vi "0814 labviewToEsp32.vi"(0 "power step  4":string, 1 "power step  3":string, 2 "power step  2":string, 3 "power step  1":string, 5 "power step  5":string, 6 "direction":string, 8 "scanspeed (um/s)":string, 9 "count":string, 10 "um":string, 11 "Ring":u16(ring) items=["Move X"=1, "Move Y"=2, "Single shot"=3, "single shot *15"=4, "energy adjustment"=5, "knife edge method"=6, "Auto mode"=7, "multiple shot"=8, "power change"=9, "shutter+move"=10, "stop"=0]) -> (4 "output":string)   [LabVIEW 2018]
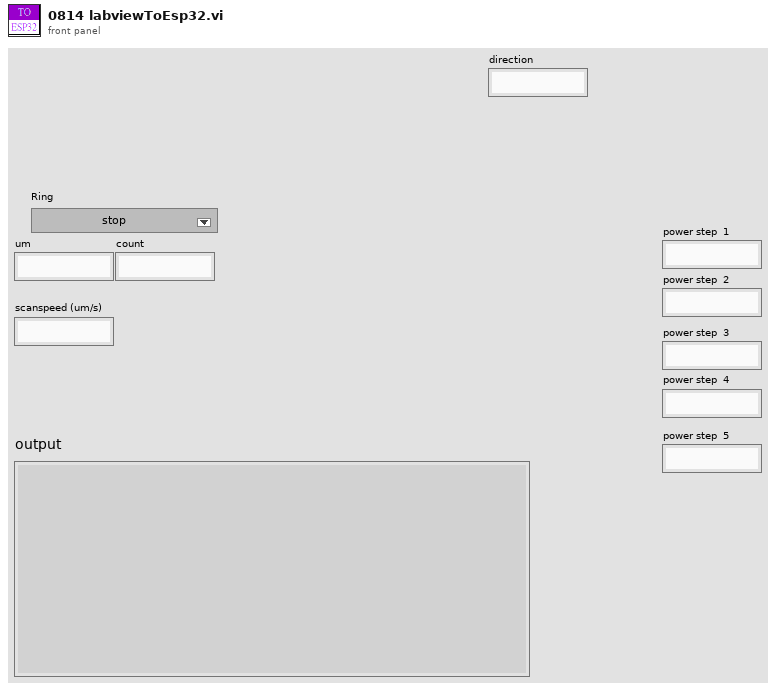
[diagram p1: front panel]
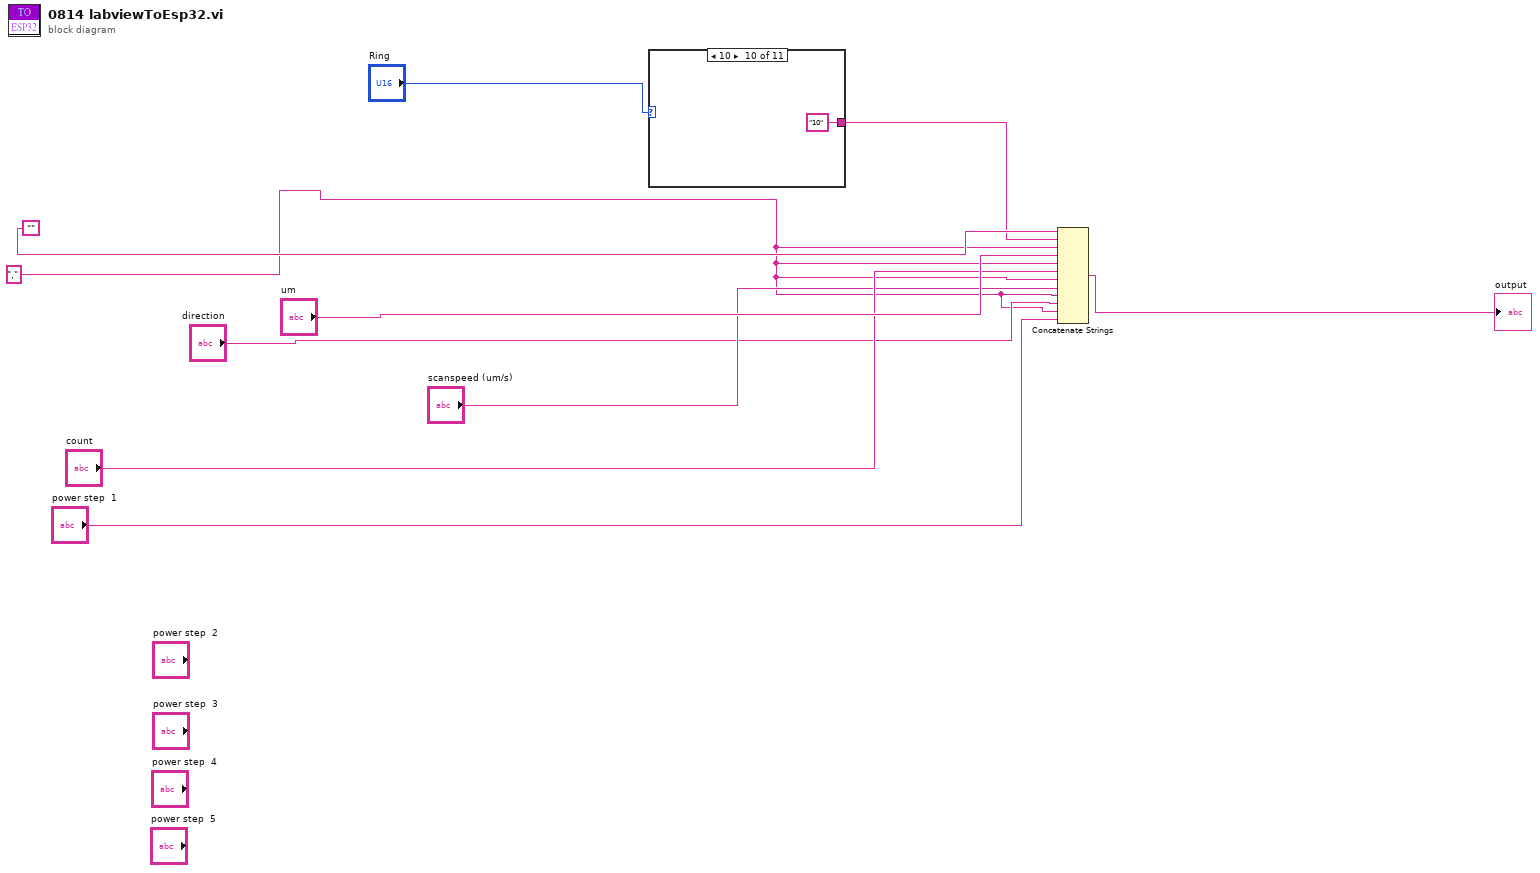
[diagram p0: block diagram]
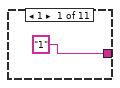
[diagram p2: hidden frame]
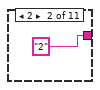
[diagram p3: hidden frame]
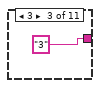
[diagram p4: hidden frame]
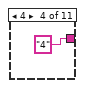
[diagram p5: hidden frame]
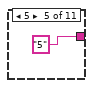
[diagram p6: hidden frame]
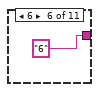
[diagram p7: hidden frame]
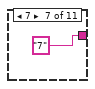
[diagram p8: hidden frame]
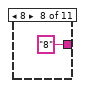
[diagram p9: hidden frame]
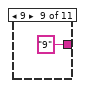
[diagram p10: hidden frame]
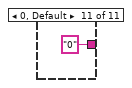
[diagram p11: hidden frame]
diagram:
  w2 = ","
  n1 = case shown="10" "Ring" {
    tunnel: ["1" "2" "3" "4" "5" "6" "7" "8" "9" "10" "0"] -> w8
    frame 1 {
    }
    frame 2 {
    }
    frame 3 {
    }
    frame 4 {
    }
    frame 5 {
    }
    frame 6 {
    }
    frame 7 {
    }
    frame 8 {
    }
    frame 9 {
    }
    frame 10 {
    }
    frame 0, Default {
    }
  }
  n2 = Concatenate Strings("", w8, w2, "um", w2, "count", w2, "scanspeed (um/s)", w2, "direction", w2, "power step  1") -> (→"output":string)
